vi "Add Sink.vi"(8 "error in (no error)":errorcluster, 9 "Sink Actor":refnum<class "Event Sink.lvclass">, 11 "Event Source in":refnum<class "Event Source.lvclass">) -> (0 "error out":errorcluster, 3 "Event Source out":refnum<class "Event Source.lvclass">)   [LabVIEW 2016, in "Event Source.lvlib" / "Event Source.lvclass"]
uses:
  Event Source.lvclass
  C:/Program Files (x86)/National Instruments/LabVIEW 2016/vi.lib/ActorFramework/Actor/Actor.lvclass
  Event Sink/Event Sink.lvclass
  Event Sink/Event Sink.lvclass/Event Sink.ctl
  Event Source.lvclass/Event Source.ctl
  <vilib>/ActorFramework/Actor/Actor.lvclass/Actor.ctl
  <vilib>/ActorFramework/Message Enqueuer/Message Enqueuer.lvclass/Message Enqueuer.ctl
  Event Sink Messages/Write Event Source Enqueuer Msg/Write Event Source Enqueuer Msg.lvclass/Write Event Source Enqueuer Msg.ctl
  Event Sink/properties/Read Name.vi
  <vilib>/ActorFramework/Message Enqueuer/Init from Existing Queue.vi
  <vilib>/ActorFramework/Message Enqueuer/Enqueue.vi
  Event Sink Messages/Write Event Source Enqueuer Msg/Write Event Source Enqueuer Msg.lvclass
  C:/Program Files (x86)/National Instruments/LabVIEW 2016/vi.lib/ActorFramework/Message/Message.lvclass
  <vilib>/Utility/LVClass/Get LV Class Name.vi
  <resource>/AFDebug/Generate Trace for Message.vi
  <vilib>/ActorFramework/Message Priority Queue/Priority Enqueue.vi
  <vilib>/ActorFramework/Message Enqueuer/Message Enqueuer.lvclass
  <vilib>/ActorFramework/Actor/Actor.lvclass
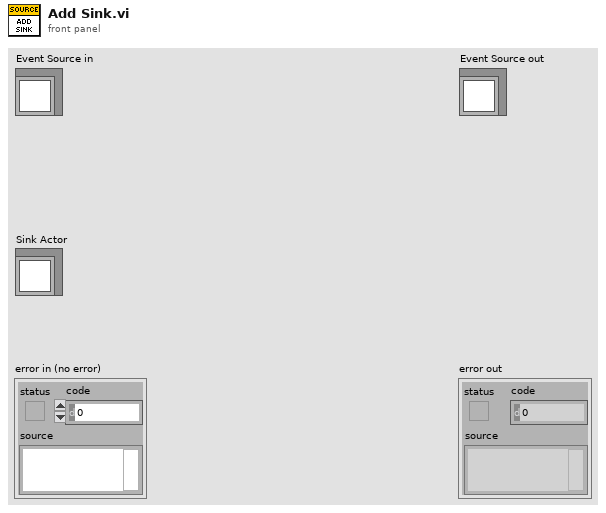
[diagram p1: front panel]
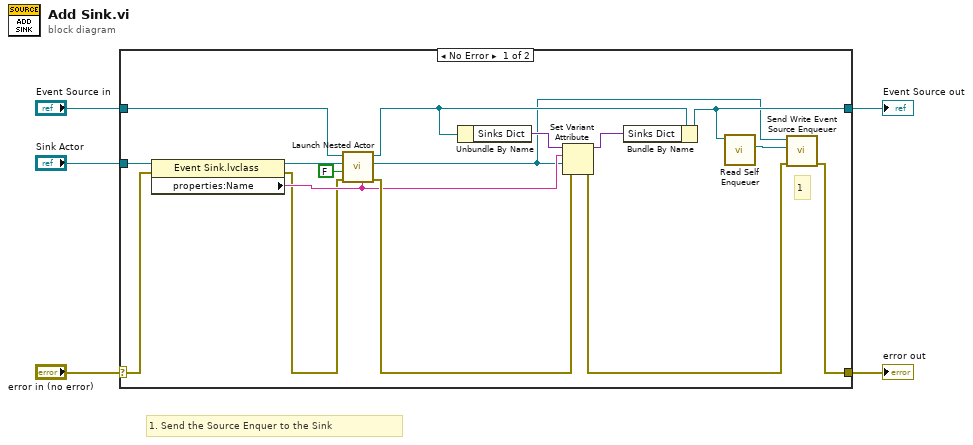
[diagram p0: block diagram]
diagram:
  # "1. Send the Source Enquer to the Sink"
  n1 = case shown="No Error" "error in (no error)" {
    selector: "error in (no error)" -> [w12 w23]
    tunnel: [w6 w23] -> w4
    tunnel: [w9 w22] -> w2
    tunnel: "Event Source in" -> [w17 w22]
    tunnel: "Sink Actor" -> [w18 _]
    frame No Error {
      # "1"
      n2 = property class="Event Sink.lvclass"(reference=w18, error in=w12) -> (reference out=w14:refnum<class "Event Sink.lvclass">, error out=w11:errorcluster, "properties:Name"=w13:string)
      n3 = call <vilib>:"Launch Nested Actor.vi"("Debug Alias"=w13, "error in (no error)"=w11, "Auto-stop? (T)"=FALSE, "Nested Actor"=w14, "Caller Actor in"=w17) -> ("error out"=w19:errorcluster, "Nested Actor's Enqueuer"=w8:refnum<class "Message Enqueuer.lvclass">, "Caller Actor out"=w16:refnum<class "Event Source.lvclass">)  [unwired: 4 in]
      n4 = Unbundle By Name(w16) -> ("Sinks Dict"=w21:variant)
      n5 = Set Variant Attribute(Variant=w21, name=w13, value=w8, error in=w19) -> (Variant out=w20:variant, error out=w7:errorcluster)  [unwired: 1 out]
      n6 = Bundle By Name(cluster=w16, "Sinks Dict"=w20) -> (w9:refnum<class "Event Source.lvclass">)
      n7 = call <vilib>:"Read Self Enqueuer.vi"("Actor"=w9) -> ("Self Enqueuer"=w10:refnum<class "Message Enqueuer.lvclass">)  [unwired: 10 in]
      n8 = call "Send Write Event Source Enqueuer.vi"("error in (no error)"=w7, "Source Actro:Message Enqueuer"=w10, "Message Enqueuer in"=w8) -> ("error out"=w6:errorcluster)  [unwired: 7 in, 1 out]
    }
    frame Error {
    }
  }
  "error out" <- w4
  "Event Source out" <- w2
